vi "Format Tag Priv.vi"(0 "Tag":string="blah", 5 "Content":string="tres") -> (4 "XML":string)   [LabVIEW 2020]
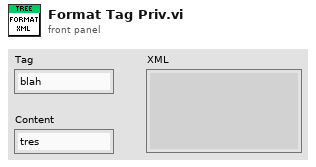
[diagram p1: front panel]
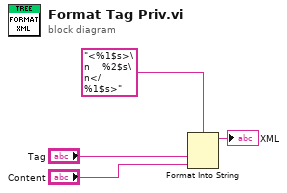
[diagram p0: block diagram]
diagram:
  n1 = Format Into String(format string="<%1$s>\n    %2$s\n</%1$s>", "Tag", "Content") -> (resulting string=→"XML":string)  [unwired: 2 in, 1 out]
